vi "Model - Get Stop.vi"(8 "error in (no error)":errorcluster, 11 "View Model":T1) -> (0 "error out":errorcluster, 2 "Stop":bool, 3 "View Model":T1)   [LabVIEW 2017]
doc: "Get actual value of Stop from DVR"
uses:
  Controls/View Model.ctl
  Controls/Shared Model.ctl
  Error Handler/Controls/Error Model.ctl
  Error Handler/Controls/Error Message.ctl
  Error Handler/Controls/Error Type.ctl
  Configuration/Controls/Config Model.ctl
  Configuration/Controls/Config DB Message.ctl
  Configuration/Controls/Config DB Command.ctl
  Configuration/Controls/Config DB Overhead.ctl
  Configuration/Controls/Config DB Record.ctl
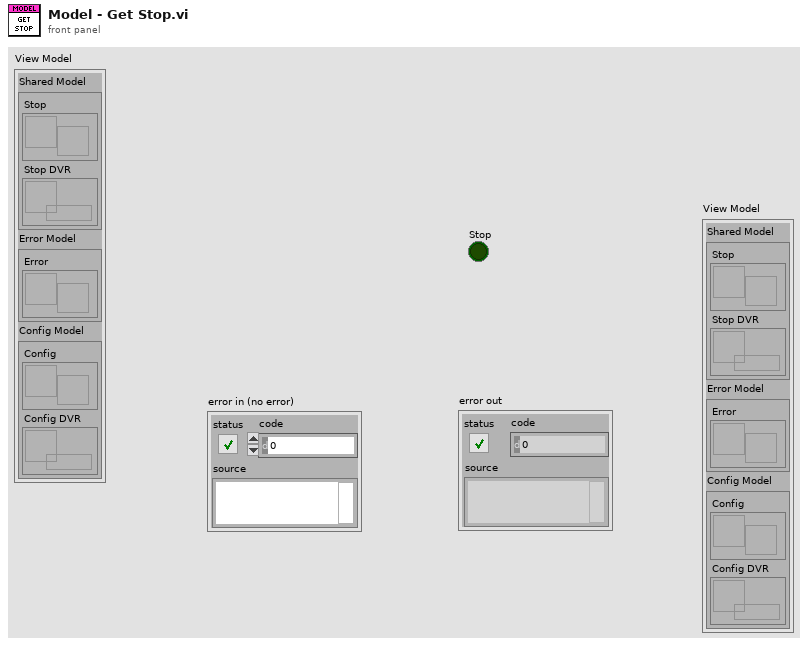
[diagram p1: front panel]
types:
  T1 = typedef "View Model.ctl" = cluster{"Shared Model":T2, "Error Model":T3, "Config Model":T4}
  T2 = typedef "Shared Model.ctl" = cluster{"Stop":refnum<user-event>, "Stop DVR":refnum<data-value>}
  T3 = typedef "Error Model.ctl" = cluster{"Error":refnum<user-event>}
  T4 = typedef "Config Model.ctl" = cluster{"Config":refnum<user-event>, "Config DVR":refnum<data-value>}
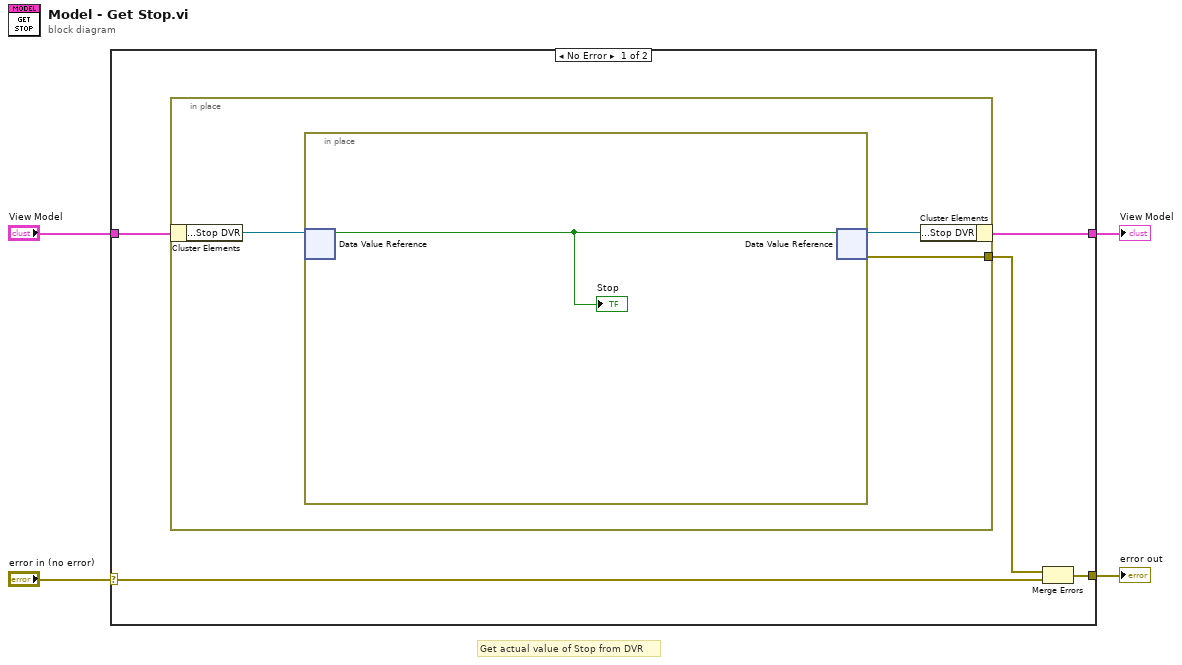
[diagram p0: block diagram]
diagram:
  # "Get actual value of Stop from DVR"
  n1 = case shown="No Error" "error in (no error)" {
    selector: "error in (no error)" -> [w7 w15]
    tunnel: "View Model" -> [w9 w14]
    tunnel: [w6 w15] -> w2
    tunnel: [w5 w14] -> w1
    frame No Error {
      n2 = in-place {
        in-place-border: [w10] -> w8
        n3 = in-place-cluster #1(w9) -> ("Shared Model.Stop DVR"=w12:refnum<data-value>)
        n4 = in-place {
          n5 = in-place-dvr #2(w12) -> (w13:bool)  [unwired: 1 out]
          "Stop" <- w13
          n6 = in-place-dvr #2(w13) -> (w11:refnum<data-value>, w10:errorcluster)
        }
        n7 = in-place-cluster #1("Shared Model.Stop DVR"=w11) -> (w5:T1)
      }
      n8 = Merge Errors(w8, w7) -> (w6:errorcluster)
    }
    frame Error {
    }
  }
  "View Model" <- w1
  "error out" <- w2
